vi "Set Magnet.vi"(4 "Axis":T1, 6 "Mode":T2, 8 "error in (no error)":errorcluster, 9 "Target Rate (T/min)":dbl, 10 "Target Field (T)":dbl, 11 "Instrument.Cryostat in":refnum<class "Instrument.VNA.lvclass">) -> (0 "error out":errorcluster, 3 "Instrument.Cryostat out":refnum<class "Instrument.VNA.lvclass">)   [LabVIEW 2016, in "Instrument.VNA.lvclass"]
uses:
  Instrument.VNA.lvclass
  Typedefs/Magnet Mode--Enum.ctl
  Typedefs/Magnet Axis--Enum.ctl
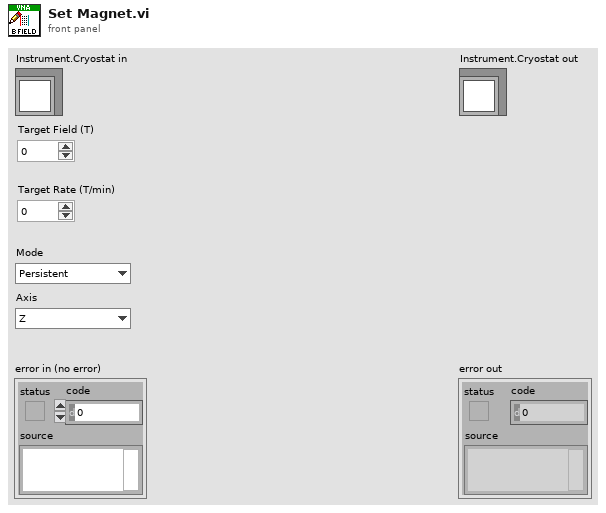
[diagram p1: front panel]
types:
  T1 = typedef "Instrument.VNA.lvclass/Magnet Axis--Enum.ctl" = enum16{"Z", "X", "Y"}
  T2 = typedef "Instrument.VNA.lvclass/Magnet Mode--Enum.ctl" = enum16{"Persistent", "Driven"}
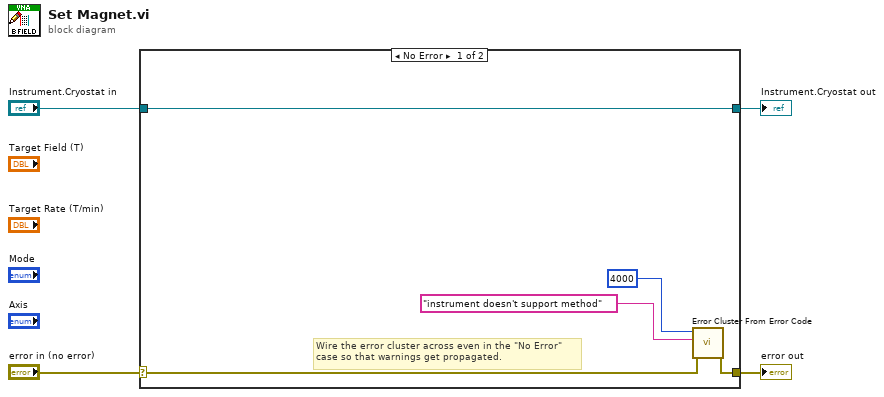
[diagram p0: block diagram]
diagram:
  n1 = case shown="No Error" "error in (no error)" {
    selector: "error in (no error)" -> [w6 w11]
    tunnel: [w5 w11] -> w3
    tunnel: [w9 w10] -> w1
    tunnel: "Instrument.Cryostat in" -> [w9 w10]
    frame No Error {
      # "Wire the error cluster across even in the \"No Error\"\ncase so that warnings get propagated."
      n2 = call <vilib>:"Error Cluster From Error Code.vi"("error in (no error)"=w6, "error message (\"\")"="instrument doesn't support method" ("error message (\"\")"), "error code (0)"=4000) -> ("error out"=w5:errorcluster)  [unwired: 6 in]
    }
    frame Error {
    }
  }
  "error out" <- w3
  "Instrument.Cryostat out" <- w1
